vi "write_fifo.vi"(8 "input ready?":bool, 10 "data":u64, 11 "on-board buffer in":T2) -> (3 "on-board buffer out":T2, 4 "write-to-FIFO status":T1, 6 "FIFO full?":bool)   [LabVIEW 2010]
uses:
  OnBoardBuffer/OnBoardBuffer.ctl
  write-to-fifo_status.ctl
  <vilib>/rvi/DataTransferAndStorage/Container/XNode/niFpgaContainer.xnode
  <vilib>/rvi/DataTransferAndStorage/Container/Common/niFpgaContainerMethod.ctl
  <vilib>/rvi/DataTransferAndStorage/Container/Common/niFpgaTransferTypeControl.ctl
  <vilib>/rvi/interface/RandomDataEmulation/nirviRandomDataFPGAFIFO.vi
  <vilib>/rvi/interface/RandomDataEmulation/niFpgaRandomDataHandleErrors.vi
  OnBoardBuffer/OnBoardBuffer.lvlib
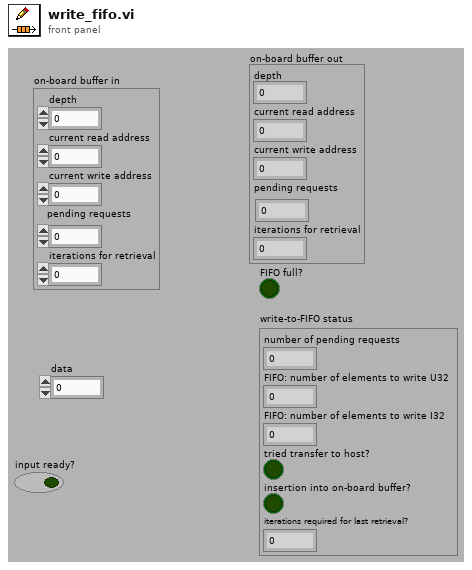
[diagram p1: front panel]
types:
  T1 = typedef "write-to-fifo_status.ctl" = cluster{"number of pending requests":i32, "FIFO: number of elements to write U32":u32, "FIFO: number of elements to write I32":i32, "tried transfer to host?":bool, "insertion into on-board buffer?":bool, "iterations required for last retrieval?":u32}
  T2 = typedef "OnBoardBuffer.lvlib/OnBoardBuffer.ctl" = cluster{"depth":u32, "current read address":u32, "current write address":u32, "pending requests":u32, "iterations for retrieval":u32}
  T3 = typedef "niFpgaContainerMethod.ctl" = enum16{"<none>", "write", "read", "clear", "getNumberOfElementsToWrite", "getNumberOfElementsToRead", "enable", "disable", "flushAndDisable", "getStreamState", "readA", "readB", "dramWrite", "dramWriteWithByteEnables", "dramRequestData", "dramRetrieveData"}
  T4 = typedef "niFpgaTransferTypeControl.ctl" = enum16{"Target-Scoped", "Host to Target - DMA", "Target to Host - DMA", "Peer to Peer Reader", "Peer to Peer Writer", "Bidirectional"}
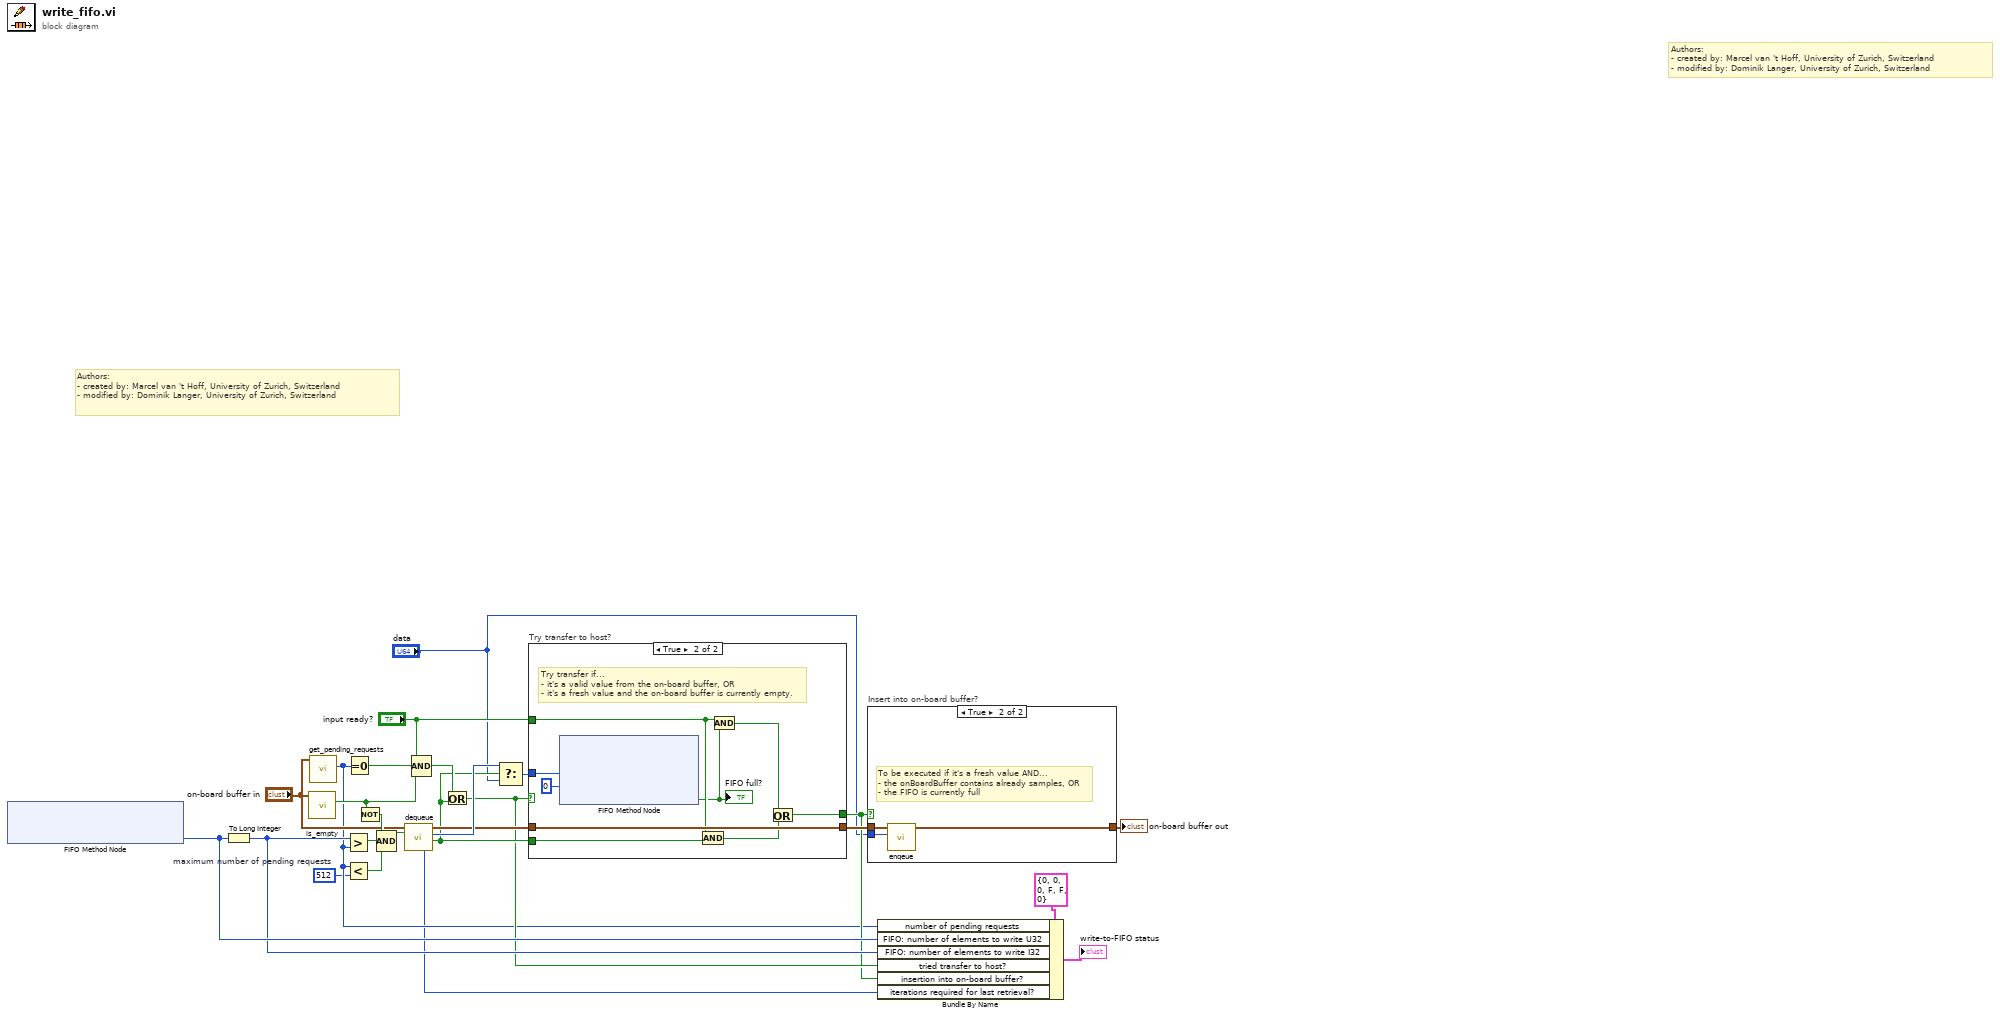
[diagram p0: block diagram]
diagram:
  w4 = 512  # maximum number of pending requests
  # "Authors: \n- created by: Marcel van 't Hoff, University of Zurich, Switzerland\n- modified by: Dominik Langer, University of Zurich, Switzerland"
  # "Authors: \n- created by: Marcel van 't Hoff, University of Zurich, Switzerland\n- modified by: Dominik Langer, University of Zurich, Switzerland"
  n1 = xnode ("FIFO Method Node")() -> ("Number of Elements to Write"=w9:u32)  [unwired: 1 in, 1 out]
  n2 = To Long Integer(number=w9) -> (32bit integer=w8:i32)
  n3 = call "is_empty.vi"("on-board buffer in"="on-board buffer in") -> ("is empty?"=w17:bool)  [unwired: 10 in]
  n4 = call "get_pending_requests.vi"("on-board buffer in"="on-board buffer in") -> ("number of pending requests"=w5:i32)  [unwired: 10 in]
  n5 = Greater?(x=w8, y=w5) -> (0:w15:bool)
  n6 = Less?(x=w5, y=w4) -> (x < y?=w3:bool)
  n7 = Equal To 0?(x=w5) -> (x = 0?=w12:bool)
  n8 = Not(x=w17) -> (.not. x?=w16:bool)
  n9 = Compound Arithmetic op=AND(w16, w15, w3) -> (w14:bool)
  n10 = call "dequeue.vi"("make request?"=w14, "on-board buffer in"="on-board buffer in") -> ("output valid?"=w18:bool, "data"=w23:u64, "on-board buffer out"=w21:T2, "iterations required for last retrieval"=w2:u32)  [unwired: 6 in]
  n11 = Compound Arithmetic op=AND("input ready?", w12, w17) -> (w24:bool)
  n12 = Or(x=w24, y=w18) -> (x .or. y?=w7:bool)
  n13 = Select(t=w23, s=w18, f="data") -> (s? t:f=w22:u64)
  n14 = case "Try transfer to host?" shown="True" w7 {
    tunnel: w22 -> [_ w35]
    tunnel: [w27 w29] -> w6
    tunnel: "input ready?" -> [w27 w32]
    tunnel: w21 -> [w26 w34]
    tunnel: [w26 w34] -> w20
    tunnel: w18 -> [_ w33]
    frame False {
    }
    frame True {
      # "Try transfer if...\n- it's a valid value from the on-board buffer, OR\n- it's a fresh value and the on-board buffer is currently empty."
      n15 = xnode ("FIFO Method Node")("Element"=w35, "Timeout"=0) -> ("Timed Out?"=w28:bool)  [unwired: 1 in, 1 out]
      "FIFO full?" <- w28
      n16 = And(x=w32, y=w33) -> (x .and. y?=w31:bool)
      n17 = And(x=w32, y=w28) -> (x .and. y?=w30:bool)
      n18 = Or(x=w30, y=w31) -> (x .or. y?=w29:bool)
    }
  }
  n19 = case "Insert into on-board buffer?" shown="True" w6 {
    tunnel: [w65 w68] -> w25
    tunnel: w20 -> [w65 w67]
    tunnel: "data" -> [_ w66]
    frame False {
    }
    frame True {
      # "To be executed if it's a fresh value AND...\n- the onBoardBuffer contains already samples, OR\n- the FIFO is currently full"
      n20 = call "enqeue.vi"("data"=w66, "on-board buffer in"=w67) -> ("on-board buffer out"=w68:T2)  [unwired: 9 in]
    }
  }
  "on-board buffer out" <- w25
  n21 = Bundle By Name(cluster=T1 {"number of pending requests"=0, "FIFO: number of elements to write U32"=0, "FIFO: number of elements to write I32"=0, "tried transfer to host?"=FALSE, "insertion into on-board buffer?"=FALSE, "iterations required for last retrieval?"=0} ("write-to-FIFO status"), "number of pending requests"=w5, "FIFO: number of elements to write U32"=w9, "FIFO: number of elements to write I32"=w8, "tried transfer to host?"=w7, "insertion into on-board buffer?"=w6, "iterations required for last retrieval?"=w2) -> (→"write-to-FIFO status":T1)
